vi "DataGraph_UpdateInfo.vi"(8 "error in (no error)":errorcluster, 10 "Information":variant, 11 "Info_Listbox":refnum<vi>) -> (0 "error out":errorcluster)   [LabVIEW 2018, in "DataGraphXControl.xctl"]
uses:
  DataGraphXControl.xctl
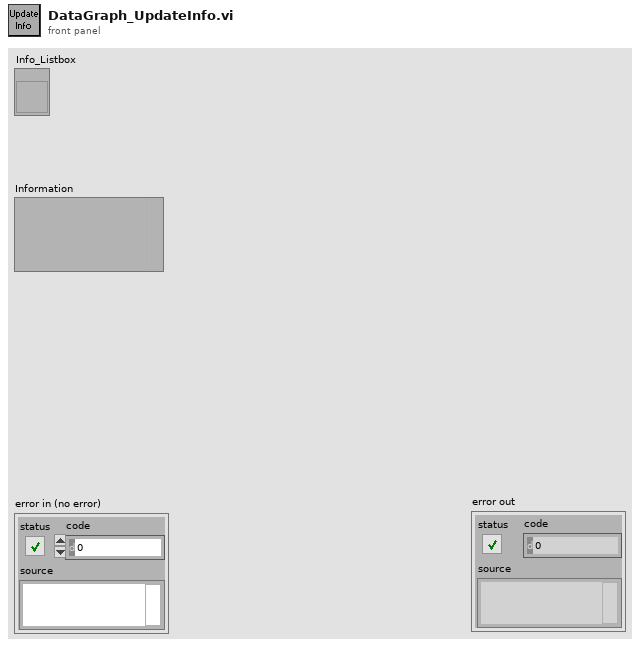
[diagram p1: front panel]
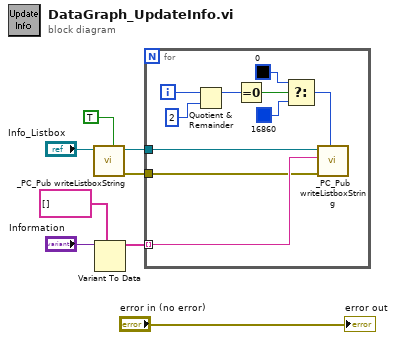
[diagram p0: block diagram]
diagram:
  n1 = call "_PC_Pub writeListboxString.vi"("Reset (F)"=TRUE, "Listbox Ref Input"="Info_Listbox") -> ("error out"=w1:errorcluster, "Listbox Ref Output"=w2:refnum<vi>)  [unwired: 8 in]
  n2 = Variant To Data(type=string[] [], Variant="Information") -> (data=w6:string[])  [unwired: 1 in, 1 out]
  n3 = for {
    tunnel: w6 -> [w10] mode=indexing
    tunnel: w2 -> [w18]
    tunnel: w1 -> [w9]
    i -> [w12]
    n4 = Quotient & Remainder(x=w12, y=2) -> (x-y*floor(x/y)=w16:i32)  [unwired: 1 out]
    n5 = Equal To 0?(x=w16) -> (x = 0?=w15:bool)
    n6 = Select(t=u32 0, s=w15, f=u32 16860) -> (s? t:f=w11:u32)
    n7 = call "_PC_Pub writeListboxString.vi"("String Color"=w11, "error in (no error)"=w9, "update_Str"=w10, "Listbox Ref Input"=w18) -> ()  [unwired: 6 in, 2 out]
  }
  "error out" <- "error in (no error)"
